vi "agilent_test_unit.vi"() -> ()   [LabVIEW 2010]
panel:
  in  "stop":bool
  out "Voltage 2 StandDev":dbl
  out "Voltage 1 StandDev":dbl
  out "Voltage 1":dbl
  out "Voltage 2":dbl
  in  "Thermal Coeffients Path":path
  in  "Agilent Port":refnum<visa-resource-name>="COM5"
  in  "voltage channels":string caption="(csv)"
  out "Room Temp":dbl
  out "Burette Temp 1":dbl
  out "Acid Temp":dbl
  out "Cell Temp":dbl
  out "Burette Temp 2":dbl
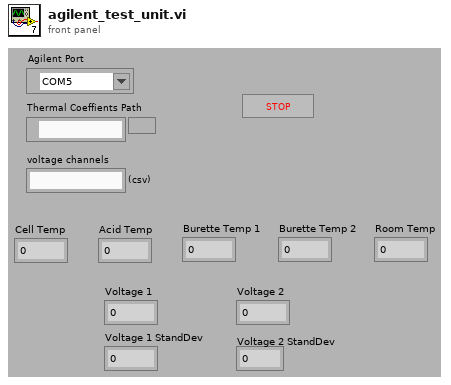
[diagram p1: front panel]
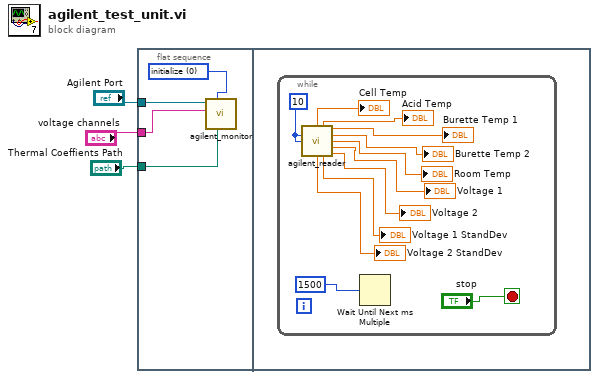
[diagram p0: block diagram]
diagram:
  n1 = flat-sequence {
    tunnel: "Agilent Port" -> [w6]
    tunnel: "Thermal Coeffients Path" -> [w5]
    tunnel: "voltage channels" -> [w4]
    frame #0 {
      w7 = u8 0 items=["initialize", "read"] ("Action")
      n2 = call "agilent_monitor.vi"("Thermal Coefficient Path"=w5, "Action"=w7, "voltage channels (csv)"=w4, "Agilent Port In"=w6) -> ()  [unwired: 5 in, 3 out]
    }
    frame #1 {
      n3 = while {
        stop <- "stop" stop-if-true
        w17 = 10
        n4 = call "agilent_reader.vi"("Voltage Readings"=w17, "Temperature Readings"=w17) -> ("Cell Temp"=→"Cell Temp":dbl, "Acid Temp"=→"Acid Temp":dbl, "Burette Temp 1"=→"Burette Temp 1":dbl, "Burette Temp 2"=→"Burette Temp 2":dbl, "Room Temp"=→"Room Temp":dbl, "Voltage 1"=→"Voltage 1":dbl, "Voltage 2 StandDev"=→"Voltage 2 StandDev":dbl, "Average Voltage"=→"Voltage 1 StandDev":dbl, "Voltage 2"=→"Voltage 2":dbl)  [unwired: 2 in, 3 out]
        n5 = Wait Until Next ms Multiple(millisecond multiple=1500) -> ()  [unwired: 1 out]
      }
    }
  }
